vi "DSF.Memory.Cache.Framework.Get Plugin Caches.vi"(8 "error in (no error)":errorcluster, 11 "Framework Cache in":refnum<class "DSF.Memory.Cache.Framework.lvclass">) -> (0 "error out":errorcluster, 2 "Plugin Caches":refnum<class "DSF.Memory.Cache.Plugin.lvclass">[](array[class]), 3 "Framework Cache out":refnum<class "DSF.Memory.Cache.Framework.lvclass">)   [LabVIEW 2016, in "DSF.Memory.lvlib" / "DSF.Memory.Cache.Framework.lvclass"]
uses:
  DSF.Memory.Cache.Framework.lvclass
  DSF.Memory.Cache.Plugin.lvclass
  DSF.Memory.Cache.Framework.lvclass/DSF.Memory.Cache.Framework.ctl
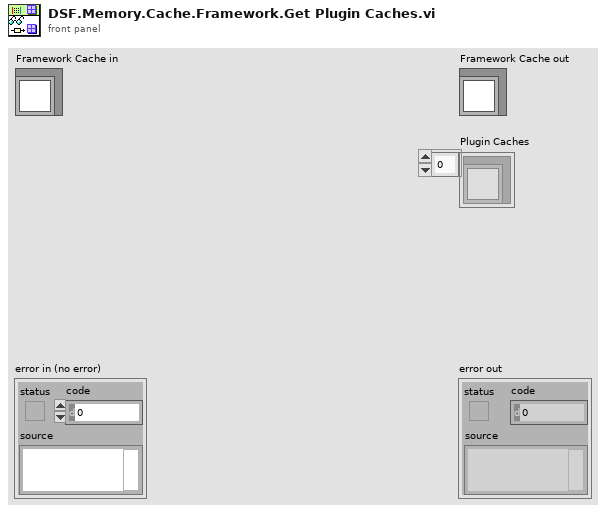
[diagram p1: front panel]
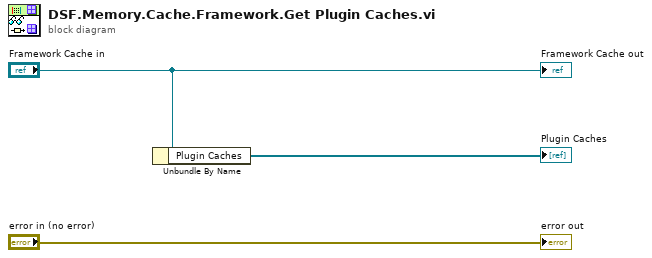
[diagram p0: block diagram]
diagram:
  n1 = Unbundle By Name("Framework Cache in") -> ("Plugin Caches"=→"Plugin Caches":refnum<class "DSF.Memory.Cache.Plugin.lvclass">[])
  "error out" <- "error in (no error)"
  "Framework Cache out" <- "Framework Cache in"
